vi "Math-FFTinv dB,degrees to x(t).vi"(8 "Nyquist Freq. Phase (degrees)":dbl format="%.2f", 9 "Nyquist Freq. Mag (rms dB)":dbl=-300.0 format="%.2f", 10 "+Freq Phase of FFT (degrees)":dbl[](array[numeric]) format="%.2f", 11 "+Freq. Mag of FFT (rms dB)":dbl[](array[numeric]) format="%.2f") -> (3 "X(t)":dbl[](array[numeric]) format="%.2f", 4 "error":i32)   [LabVIEW 2020]
uses:
  <vilib>/Analysis/2dsp.llb/Inverse Real FFT.vi
  <vilib>/Analysis/NI_AALPro.lvlib
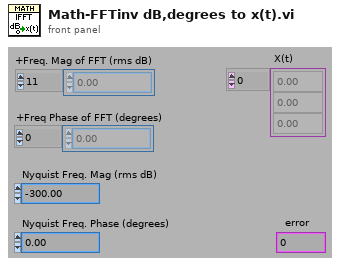
[diagram p1: front panel]
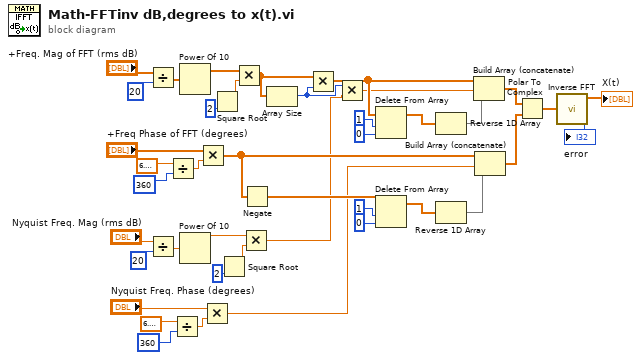
[diagram p0: block diagram]
diagram:
  n1 = Divide(x="+Freq. Mag of FFT (rms dB)", y=20) -> (x/y=w9:dbl[])
  n2 = Divide(x="Nyquist Freq. Mag (rms dB)", y=20) -> (x/y=w19:dbl)
  n3 = Divide(x=6.283185307179586, y=360) -> (x/y=w36:dbl)
  n4 = Divide(x=6.283185307179586, y=360) -> (x/y=w17:dbl)
  n5 = Power Of 10(x=w9) -> (10^x=w6:dbl[])
  n6 = Power Of 10(x=w19) -> (10^x=w2:dbl)
  n7 = Multiply(x="+Freq Phase of FFT (degrees)", y=w36) -> (x*y=w33:dbl[])
  n8 = Multiply(x="Nyquist Freq. Phase (degrees)", y=w17) -> (x*y=w13:dbl)
  n9 = Square Root(x=2) -> (sqrt(x)=w8:dbl)
  n10 = Square Root(x=2) -> (sqrt(x)=w4:dbl)
  n11 = Multiply(x=w6, y=w8) -> (x*y=w5:dbl[])
  n12 = Multiply(x=w2, y=w4) -> (x*y=w1:dbl)
  n13 = Negate(x=w33) -> (-x=w23:dbl[])
  n14 = Array Size(array=w5) -> (size(s)=w10:i32)
  n15 = Multiply(x=w5, y=w10) -> (x*y=w22:dbl[])
  n16 = Multiply(x=w10, y=w1) -> (x*y=w11:dbl)
  n17 = Delete From Array(array=w22, length=1, index=0) -> (array with subset deleted=w29:dbl[])  [unwired: 1 out]
  n18 = Delete From Array(array=w23, length=1, index=0) -> (array with subset deleted=w26:dbl[])  [unwired: 1 out]
  n19 = Reverse 1D Array(array=w29) -> (reversed array=w21:dbl[])
  n20 = Reverse 1D Array(array=w26) -> (reversed array=w20:dbl[])
  n21 = Build Array (concatenate)(w22, w11, w21) -> (w38:dbl[])
  n22 = Build Array (concatenate)(w33, w13, w20) -> (w37:dbl[])
  n23 = Polar To Complex(1:w37, 2:w38) -> (0:w40:cdb[])
  n24 = call-poly <vilib>:"Inverse FFT.vi"("FFT {X}"=w40) -> ("error"=→"error":i32, "X"=→"X(t)":dbl[])  [unwired: 9 in]
